vi "ReadAll.vi"(8 "error in (no error)":errorcluster, 9 "timeout":u32=5000, 10 "value":string="ok", 11 "VISA resource in":refnum<visa-resource-name>) -> (0 "error out":errorcluster, 1 "timeout?":bool, 2 "result":string, 3 "VISA resource out":refnum<visa-resource-name>)   [LabVIEW 2014]
panel:
  out "start time":u32
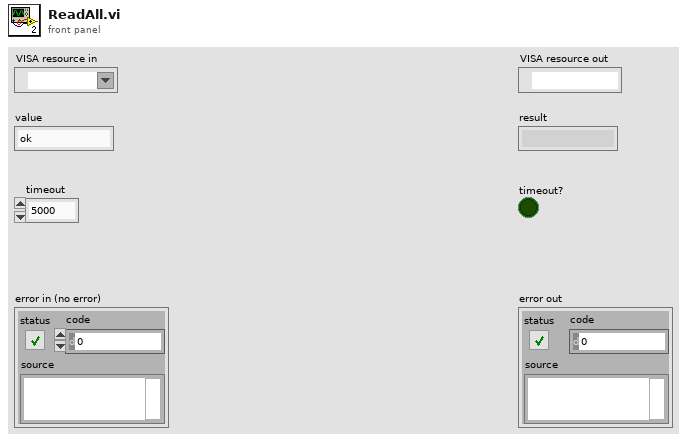
[diagram p1: front panel]
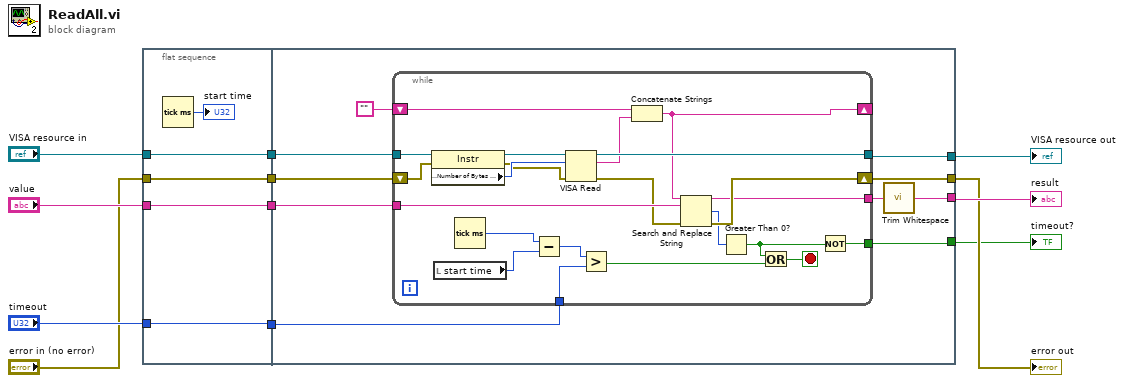
[diagram p0: block diagram]
diagram:
  n1 = flat-sequence {
    tunnel: "VISA resource in" -> [w17]
    tunnel: [w17] -> w9
    tunnel: [w15] -> w8
    tunnel: "timeout" -> [w15]
    tunnel: "value" -> [w14]
    tunnel: [w14] -> w5
    tunnel: "error in (no error)" -> [w13]
    tunnel: [w13] -> w4
    tunnel: [w18] -> w12
    tunnel: [w25] -> w10
    tunnel: w9 -> [w26]
    tunnel: w8 -> [w24]
    tunnel: w5 -> [w23]
    tunnel: w4 -> [w22]
    tunnel: [w21] -> w2
    tunnel: [w20] -> w1
    frame #0 {
      n2 = Tick Count (ms)() -> (millisecond timer value=→"start time":u32)
    }
    frame #1 {
      n3 = while {
        tunnel: w26 -> [w45]
        tunnel: [w49] -> w25
        shift-right: [w35] -> _
        shift-left: "" -> [w48]
        tunnel: w24 -> [w39]
        tunnel: w23 -> [w34]
        shift-right: [w32] -> w21
        shift-left: w22 -> [w36]
        tunnel: [w29] -> w20
        tunnel: [w28] -> w19
        stop <- w37 stop-if-true
        n4 = property class="Instr"(reference=w45, error in=w36) -> (reference out=w46:refnum<visa-resource-name>, error out=w43:errorcluster, "Serial Settings:Number of Bytes at Serial Port"=w44:u32)
        n5 = local read "start time"() -> (w41:u32)
        n6 = Tick Count (ms)() -> (millisecond timer value=w42:u32)
        n7 = Subtract(x=w42, y=w41) -> (x-y=w40:u32)
        n8 = VISA Read(VISA resource name=w46, byte count=w44, error in (no error)=w43) -> (VISA resource name out=w49:refnum<visa-resource-name>, read buffer=w47:string, error out=w33:errorcluster)  [unwired: 1 out]
        n9 = Greater?(x=w40, y=w39) -> (0:w38:bool)
        n10 = Concatenate Strings(w48, w47) -> (w35:string)
        n11 = Search and Replace String(input string=w35, search string=w34, error in=w33) -> (result string=w28:string, number of replacements=w31:i32, error out=w32:errorcluster)  [unwired: 5 in, 1 out]
        n12 = Greater Than 0?(x=w31) -> (x > 0?=w30:bool)
        n13 = Or(x=w30, y=w38) -> (x .or. y?=w37:bool)
        n14 = Not(x=w30) -> (.not. x?=w29:bool)
      }
      n15 = call <vilib>:"Trim Whitespace.vi"("string"=w19) -> ("trimmed string"=w18:string)  [unwired: 1 in]
    }
  }
  "result" <- w12
  "VISA resource out" <- w10
  "error out" <- w2
  "timeout?" <- w1
